vi "Read Port.vi"(8 "error in (no error)":errorcluster, 9 "Port 2":u16, 10 "VISA resource name":refnum<visa-resource-name>, 11 "NXP in":refnum<class "NXP.lvclass">) -> (0 "error out":errorcluster, 1 "Array":bool[](array[boolean]), 2 "VISA resource name 2":refnum<visa-resource-name>, 3 "NXP out":refnum<class "NXP.lvclass">)   [LabVIEW 2020, in "NXP.lvclass"]
uses:
  NXP.lvclass
panel:
  out "String 2":string
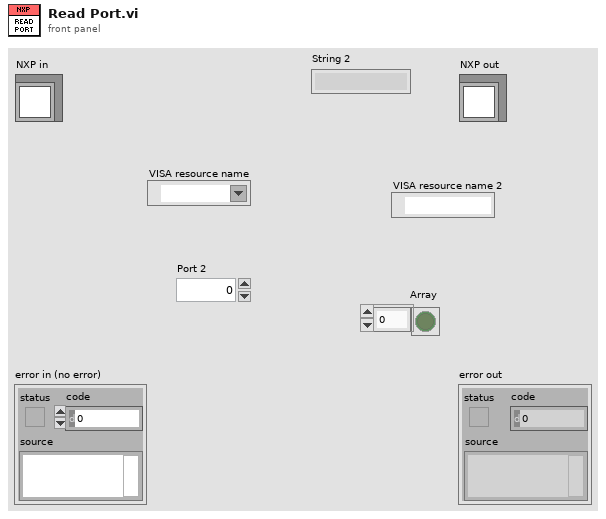
[diagram p1: front panel]
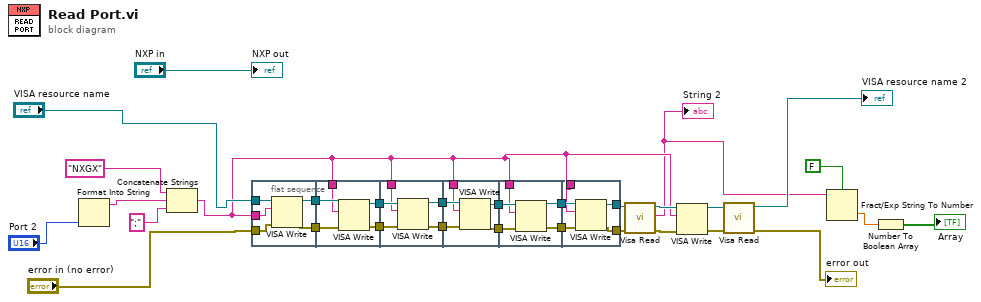
[diagram p0: block diagram]
diagram:
  n1 = Format Into String("Port 2") -> (resulting string=w29:string)  [unwired: 3 in, 1 out]
  n2 = Concatenate Strings("NXGX" ("string"), w29, ";" ("string")) -> (w2:string)
  n3 = flat-sequence {
    tunnel: "VISA resource name" -> [w35]
    tunnel: w2 -> [w34]
    tunnel: "error in (no error)" -> [w33]
    tunnel: [w32] -> w14
    tunnel: [w31] -> w13
    tunnel: w14 -> [w40]
    tunnel: w13 -> [w39]
    tunnel: [w38] -> w12
    tunnel: [w37] -> w11
    tunnel: w2 -> [w36]
    tunnel: w12 -> [w45]
    tunnel: w11 -> [w44]
    tunnel: [w43] -> w10
    tunnel: [w42] -> w9
    tunnel: w2 -> [w41]
    tunnel: [w50] -> w20
    tunnel: [w49] -> w19
    tunnel: w10 -> [w48]
    tunnel: w9 -> [w47]
    tunnel: w2 -> [w46]
    tunnel: w20 -> [w55]
    tunnel: w19 -> [w54]
    tunnel: [w53] -> w18
    tunnel: [w52] -> w17
    tunnel: w2 -> [w51]
    tunnel: w18 -> [w60]
    tunnel: w17 -> [w59]
    tunnel: w2 -> [w58]
    tunnel: [w57] -> w6
    tunnel: [w56] -> w5
    frame #0 {
      n4 = VISA Write(VISA resource name=w35, write buffer=w34, error in (no error)=w33) -> (VISA resource name out=w32:refnum<visa-resource-name>, error out=w31:errorcluster)  [unwired: 1 out]
    }
    frame #1 {
      n5 = VISA Write(VISA resource name=w40, write buffer=w36, error in (no error)=w39) -> (VISA resource name out=w38:refnum<visa-resource-name>, error out=w37:errorcluster)  [unwired: 1 out]
    }
    frame #2 {
      n6 = VISA Write(VISA resource name=w45, write buffer=w41, error in (no error)=w44) -> (VISA resource name out=w43:refnum<visa-resource-name>, error out=w42:errorcluster)  [unwired: 1 out]
    }
    frame #3 {
      n7 = VISA Write(VISA resource name=w48, write buffer=w46, error in (no error)=w47) -> (VISA resource name out=w49:refnum<visa-resource-name>, error out=w50:errorcluster)  [unwired: 1 out]
    }
    frame #4 {
      n8 = VISA Write(VISA resource name=w54, write buffer=w51, error in (no error)=w55) -> (VISA resource name out=w52:refnum<visa-resource-name>, error out=w53:errorcluster)  [unwired: 1 out]
    }
    frame #5 {
      n9 = VISA Write(VISA resource name=w59, write buffer=w58, error in (no error)=w60) -> (VISA resource name out=w57:refnum<visa-resource-name>, error out=w56:errorcluster)  [unwired: 1 out]
    }
  }
  n10 = call "Visa Read.vi"("error in (no error)"=w5, "VISA Refnum in"=w6) -> ("error out"=w8:errorcluster, "String 2"=w1:string, "VISA Refnum out"=w7:refnum<visa-resource-name>)  [unwired: 7 in]
  "String 2" <- w1
  n11 = VISA Write(VISA resource name=w7, write buffer=w2, error in (no error)=w8) -> (VISA resource name out=w4:refnum<visa-resource-name>, error out=w3:errorcluster)  [unwired: 1 out]
  n12 = call "Visa Read.vi"("error in (no error)"=w3, "VISA Refnum in"=w4) -> ("error out"=→"error out":errorcluster, "VISA Refnum out"=→"VISA resource name 2":refnum<visa-resource-name>)  [unwired: 7 in, 1 out]
  n13 = Fract/Exp String To Number(use system decimal point (T)=FALSE, string=w1) -> (number=w23:dbl)  [unwired: 2 in, 1 out]
  n14 = Number To Boolean Array(number=w23) -> (Boolean array=→"Array":bool[])
  "NXP out" <- "NXP in"
